vi "External Transition.vi"(8 "error in (no error)":errorcluster, 9 "Target State":refnum<class "State.lvclass">, 10 "Context in":refnum<data-value>, 11 "Nested State in":refnum<class "Nested State.lvclass">) -> (0 "error out":errorcluster, 2 "Context out":refnum<data-value>, 3 "State out":refnum<class "State.lvclass">)   [LabVIEW 2024, in "State.lvlib" / "Nested State.lvclass"]
uses:
  Nested State.lvclass
  C:/Users/ottoa/OneDrive/Desktop/working copies/stateMachineActor/src/State Machine/State/State/State.lvclass
  State/State.lvclass
  Context/Context/Context.lvclass
  Nested State.lvclass/Nested State.ctl
  C:/Users/ottoa/OneDrive/Desktop/working copies/stateMachineActor/src/State Machine/State/~State/~State.lvclass
  C:/Users/ottoa/OneDrive/Desktop/working copies/stateMachineActor/src/State Machine/State/Nested State/Nested State.lvclass
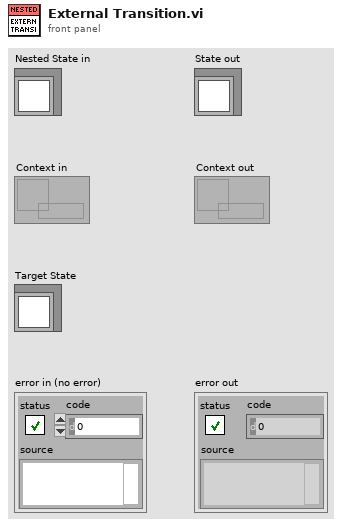
[diagram p1: front panel]
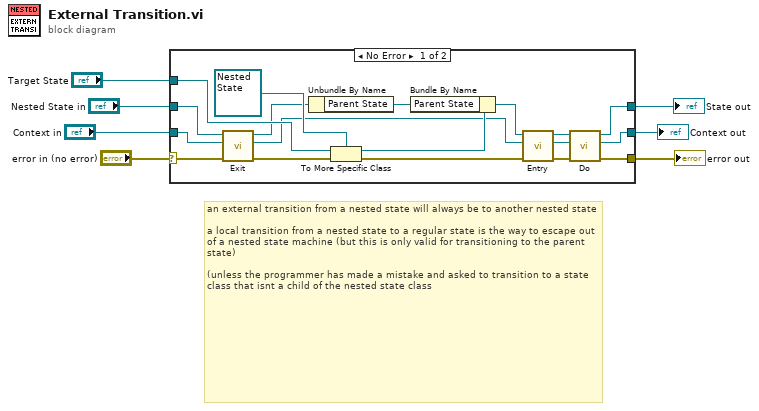
[diagram p0: block diagram]
diagram:
  # "an external transition from a nested state will always be to another nested state\n\na local transition from a nested state to a regular state is the way to escape out of a nested state machine (but this is only valid for transitioning to the parent state)\n\n(unless the programmer has made a mistake and asked to transition to a state class that isnt a child of the nested state class"
  n1 = case shown="No Error" "error in (no error)" {
    selector: "error in (no error)" -> [w8 w27]
    tunnel: "Target State" -> [w24 _]
    tunnel: "Nested State in" -> [w21 w26]
    tunnel: "Context in" -> [w20 w28]
    tunnel: [w13 w27] -> w4
    tunnel: [w12 w28] -> w3
    tunnel: [w9 w26] -> w2
    frame No Error {
      n2 = call-dynamic "Exit.vi"("error in (no error)"=w8, "Context in"=w20, "State in"=w21) -> ("error out"=w11:errorcluster, "Context out"=w14:refnum<data-value>, "State out"=w19:refnum<class "Nested State.lvclass">)  [unwired: 6 in]
      n3 = Unbundle By Name(w19) -> ("Parent State"=w22:refnum<class "State.lvclass">)
      n4 = To More Specific Class(target class=refnum<class "Nested State.lvclass"> refnum ("Nested State in"), reference=w24, error in=w11) -> (specific class reference=w23:refnum<class "Nested State.lvclass">, error out=w10:errorcluster)
      n5 = Bundle By Name(cluster=w23, "Parent State"=w22) -> (w18:refnum<class "Nested State.lvclass">)
      n6 = call-dynamic "Entry.vi"("error in (no error)"=w10, "Context in"=w14, "State in"=w18) -> ("error out"=w17:errorcluster, "Context out"=w16:refnum<data-value>, "State out"=w15:refnum<class "Nested State.lvclass">)  [unwired: 6 in]
      n7 = call-dynamic "Do.vi"("error in (no error)"=w17, "Context in"=w16, "State in"=w15) -> ("error out"=w13:errorcluster, "Context out"=w12:refnum<data-value>, "State out"=w9:refnum<class "Nested State.lvclass">)  [unwired: 6 in]
    }
    frame Error {
    }
  }
  "error out" <- w4
  "Context out" <- w3
  "State out" <- w2
